vi "ex10.vi"() -> ()   [LabVIEW 2022 SP3]
panel:
  out "Boolean":bool
  in  "String":string
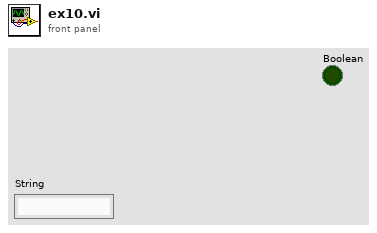
[diagram p1: front panel]
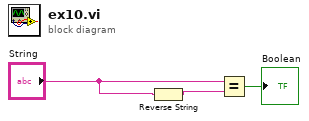
[diagram p0: block diagram]
diagram:
  n1 = Reverse String(1:"String") -> (0:w3:string)
  n2 = Equal?(x="String", y=w3) -> (x = y?=→"Boolean":bool)
